vi "VICI Reserve Pump Queue Version.vi"(8 "error in (no error)":errorcluster, 10 "Pump ID":string, 11 "VISA # in":string) -> (0 "error out":errorcluster, 2 "Loop Completed":bool, 3 "VISA # out":string)   [LabVIEW 2018, in "VICI M6 M50 Party Mode.lvlib" / "VICI Global Library.lvlib"]
uses:
  VICI Global Library.lvlib
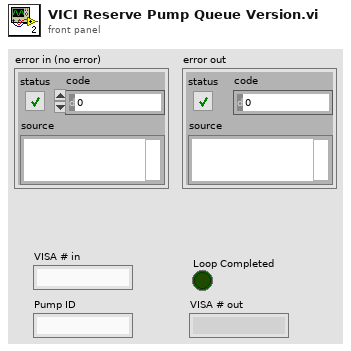
[diagram p1: front panel]
types:
  T1 = typedef "VICI M6 M50 Party Mode.lvlib/VICI Global Library.lvlib/VICI Global.ctl" = cluster{"Busy":bool, "VISA #":string, "Current Pump":string, "Current Function":string, "Pump Array":string[], "Last Success":timestamp, "ID Queue":string[]}
  T2 = cluster{"Busy":bool, "VISA #":string, "Current Pump":string, "Current Function":string, "Pump Array":string[], "Last Success":timestamp, "ID Queue":string[]}[]
  T3 = cluster{"Busy":bool, "VISA #":string, "Current Pump":string, "Current Function":string, "Pump Array":string[], "Last Success":timestamp, "ID Queue":string[]}
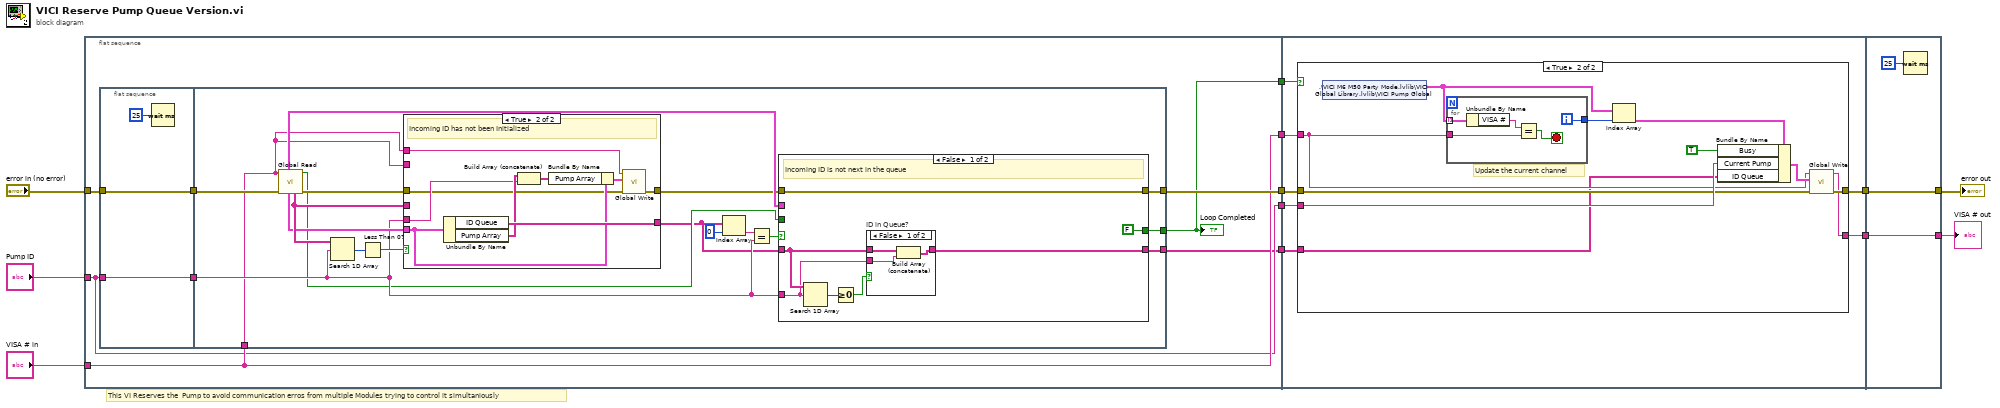
[diagram p0: block diagram]
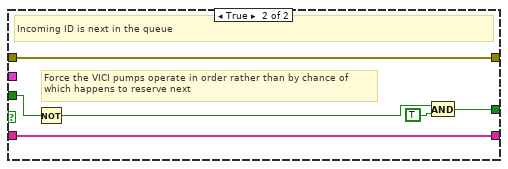
[diagram p3: hidden frame]
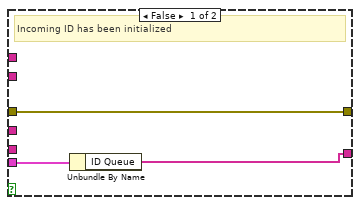
[diagram p4: hidden frame]
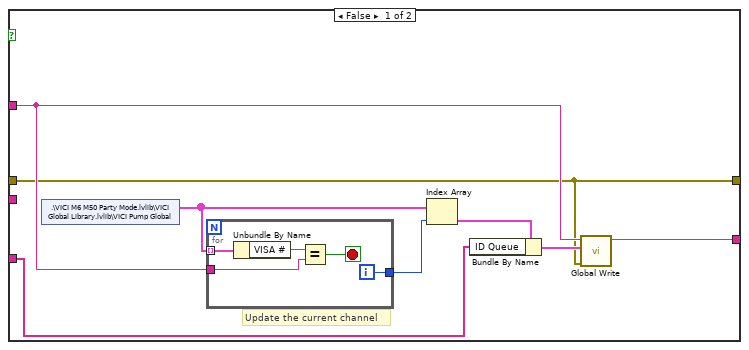
[diagram p5: hidden frame]
diagram:
  # "This VI Reserves the  Pump to avoid communication erros from multiple Modules trying to control it simultaniously"
  n1 = flat-sequence {
    tunnel: [w19] -> w12
    tunnel: [w16] -> w11
    tunnel: "error in (no error)" -> [w20]
    tunnel: [w15] -> w10
    tunnel: "Pump ID" -> [w15]
    tunnel: [w17] -> w9
    tunnel: "VISA # in" -> [w16]
    tunnel: [w13] -> w1
    tunnel: [w75] -> w8
    tunnel: w12 -> [w76]
    tunnel: w11 -> [w74]
    tunnel: w10 -> [w73]
    tunnel: [w72] -> w7
    tunnel: w9 -> [w71]
    tunnel: w1 -> [w70]
    tunnel: [w108] -> w6
    tunnel: w8 -> [w108]
    tunnel: [w106] -> w3
    tunnel: w7 -> [w106]
    frame #0 {
      n2 = flat-sequence {
        tunnel: [w23] -> w18
        tunnel: w20 -> [w23]
        tunnel: w15 -> [w21]
        tunnel: [w21] -> w14
        tunnel: [w27] -> w19
        tunnel: [w28] -> w17
        tunnel: w18 -> [w38]
        tunnel: w16 -> [w33]
        tunnel: w14 -> [w34]
        tunnel: [w26] -> w13
        frame #0 {
          n3 = Wait (ms)(milliseconds to wait=u32 25) -> ()  [unwired: 1 out]
        }
        frame #1 {
          n4 = call "Global Read.vi"("VISA #"=w33, "error in (no error)"=w38) -> ("Global for this VISA"=w35:T1, "Pump Array"=w37:string[], "Busy"=w29:bool, "error out"=w36:errorcluster)  [unwired: 2 in, 3 out]
          n5 = Search 1D Array(1D array=w37, element=w34) -> (index of element=w40:i32)  [unwired: 1 in]
          n6 = Less Than 0?(x=w40) -> (x < 0?=w39:bool)
          n7 = case shown="True" w39 {
            tunnel: w36 -> [w60 w62]
            tunnel: [w60 w61] -> w25
            tunnel: w37 -> [_ _]
            tunnel: w33 -> [_ _]
            tunnel: w34 -> [_ w67]
            tunnel: w35 -> [w59 w66]
            tunnel: [w58 w69] -> w24
            tunnel: w33 -> [_ w63]
            frame False {
              # "Incoming ID has been initialized"
              n8 = Unbundle By Name(w59) -> ("ID Queue"=w58:string[])
            }
            frame True {
              # "Incoming ID has not been Initialized"
              n9 = Unbundle By Name(w66) -> ("ID Queue"=w69:string[], "Pump Array"=w68:string[])
              n10 = Build Array (concatenate)(w68, w67) -> (w65:string[])
              n11 = Bundle By Name(cluster=w66, "Pump Array"=w65) -> (w64:T1)
              n12 = call "Global Write.vi"("error in (no error)"=w62, "VICI Global"=w64, "VISA # in"=w63) -> ("error out"=w61:errorcluster)  [unwired: 7 in, 1 out]
            }
          }
          n13 = Index Array(array=w24, index=0) -> (element=w32:string)
          n14 = Equal?(x=w32, y=w34) -> (x = y?=w31:bool)
          n15 = case shown="False" w31 {
            tunnel: w24 -> [w45 w57]
            tunnel: w34 -> [w44 _]
            tunnel: w35 -> [_ _]
            tunnel: w29 -> [_ w55]
            tunnel: [FALSE w54] -> w28
            tunnel: [w43 w53] -> w27
            tunnel: w25 -> [w43 w53]
            tunnel: [w41 w57] -> w26
            frame False {
              # "Incoming ID is not next in the queue"
              n16 = Search 1D Array(1D array=w45, element=w44) -> (index of element=w46:i32)  [unwired: 1 in]
              n17 = Greater Or Equal To 0?(x=w46) -> (x >= 0?=w42:bool)
              n18 = case "ID in Queue?" shown="False" w42 {
                tunnel: w45 -> [w50 w51]
                tunnel: w44 -> [w49 _]
                tunnel: [w48 w51] -> w41
                frame False {
                  n19 = Build Array (concatenate)(w50, w49) -> (w48:string[])
                }
                frame True {
                }
              }
            }
            frame True {
              # "Force the VICI pumps operate in order rather than by chance of\nwhich happens to reserve next"
              # "Incoming ID is next in the queue"
              n20 = Not(x=w55) -> (.not. x?=w56:bool)
              n21 = And(x=w56, y=TRUE) -> (x .and. y?=w54:bool)
            }
          }
        }
      }
      "Loop Completed" <- w17
    }
    frame #1 {
      n22 = case shown="True" w71 {
        tunnel: w76 -> [w78 w93]
        tunnel: [w78 w94] -> w75
        tunnel: w74 -> [w80 w91]
        tunnel: w73 -> [_ w97]
        tunnel: [w77 w92] -> w72
        tunnel: w70 -> [w79 w90]
        frame False {
          # "Update the current channel"
          n23 = shared-variable ".\\VICI M6 M50 Party Mode.lvlib\\VICI Global Library.lvlib\\VICI Pump Global"() -> (w83:T2)  [unwired: 1 in, 1 out]
          n24 = for {
            tunnel: w83 -> [w89] mode=indexing
            tunnel: w80 -> [w87]
            tunnel: [w85] -> w82
            i -> [w85]
            stop <- w86 stop-if-true
            n25 = Unbundle By Name(w89) -> ("VISA #"=w88:string)
            n26 = Equal?(x=w88, y=w87) -> (x = y?=w86:bool)
          }
          n27 = Index Array(array=w83, index=w82) -> (element=w84:T3)
          n28 = Bundle By Name(cluster=w84, "ID Queue"=w79) -> (w81:T3)
          n29 = call "Global Write.vi"("error in (no error)"=w78, "VICI Global"=w81, "VISA # in"=w80) -> ("VISA # out"=w77:string)  [unwired: 7 in, 1 out]
        }
        frame True {
          # "Update the current channel"
          n30 = shared-variable ".\\VICI M6 M50 Party Mode.lvlib\\VICI Global Library.lvlib\\VICI Pump Global"() -> (w98:T2)  [unwired: 1 in, 1 out]
          n31 = for {
            tunnel: w98 -> [w105] mode=indexing
            tunnel: w91 -> [w103]
            tunnel: [w101] -> w96
            i -> [w101]
            stop <- w102 stop-if-true
            n32 = Unbundle By Name(w105) -> ("VISA #"=w104:string)
            n33 = Equal?(x=w104, y=w103) -> (x = y?=w102:bool)
          }
          n34 = Index Array(array=w98, index=w96) -> (element=w99:T3)
          n35 = Bundle By Name(cluster=w99, "Busy"=TRUE, "Current Pump"=w97, "ID Queue"=w90) -> (w95:T3)
          n36 = call "Global Write.vi"("error in (no error)"=w93, "VICI Global"=w95, "VISA # in"=w91) -> ("error out"=w94:errorcluster, "VISA # out"=w92:string)  [unwired: 7 in]
        }
      }
    }
    frame #2 {
      n37 = Wait (ms)(milliseconds to wait=u32 25) -> ()  [unwired: 1 out]
    }
  }
  "error out" <- w6
  "VISA # out" <- w3
